vi "GameToIAState.vi"(8 "error in (no error)":errorcluster, 11 "Game in":refnum<class "Game.lvclass">) -> (0 "error out":errorcluster, 2 "IA State out":T1={"our_robots"=[], "enemy_robots"=[], "balls"=[], "geometry"={"line_width"=0, "field_length"=0, "field_width"=0, "boundary_width"=0, "referee_width"=0, "goal_width"=0, "goal_depth"=0, "goal_wall_width"=0, "center_circle_radius"=0, "defense_radius"=0, "defense_stretch"=0, "free_kick_from_defense_dist"=0, "penalty_spot_from_field_line_dist"=0, "penalty_line_from_spot_dist"=0}, "IA Judge"={"stage"="", "command"="", "our_goalie_id"=0.0, "enemy_goalie_id"=0.0, "command enum"=enum."Halt", "Time"=enum."Azul"}, "Received Timestamp"=timestamp(0 s since 1904-01-01), "Events"={"Touch"=FALSE, "Ball out"=FALSE, "id touch"=0.0, "Ball out of \nVision"=FALSE, "Ball inside \nGoalie area"=FALSE, "Robot not responding"=FALSE, "Robots responding status"=[1.0, 1.0, 1.0, 1.0, 1.0, 1.0], "Enemy Ball \nPossession"=FALSE, "Pass State"=FALSE, "id end of pass"=0.0, "Kick"=FALSE, "Id ini Possession"=0.0, "Ball Possesion"=FALSE, "Id Possesion"=0.0, "Direct Kick"=FALSE, "2nd Strk Ativo"=FALSE}}, 3 "Game out":refnum<class "Game.lvclass">)   [LabVIEW 2023, in "Game.lvclass"]
uses:
  Game.lvclass
  Vision_class/Old vision/SSL Detection Frame Simple Estimator Cameras VelCmd Folder/Core/AI Input.ctl
  Vision_class/Old vision/Controls/AI Robot.ctl
  Vision_class/Old vision/Controls/Functions Enum.ctl
  Vision_class/Old vision/Controls/AttackerStates.ctl
  Vision_class/Old vision/Controls/PathDests.ctl
  Vision_class/Old vision/Controls/PathDest.ctl
  Navigation/VSSNavigation/VSSAttackerStates.ctl
  Vision_class/Old vision/SSL Detection Frame Simple Estimator Cameras VelCmd Folder/Core/AI Ball.ctl
  Vision_class/Old vision/SSL Detection Frame Simple Estimator Cameras VelCmd Folder/Core/Field Size.ctl
  Vision_class/Old vision/SSL Detection Frame Simple Estimator Cameras VelCmd Folder/Core/AI Judge.ctl
  Communication_class/Paths/MessageAI_State Folder/Intel/Command Enum.ctl
  Vision_class/Old vision/SSL Detection Frame Simple Estimator Cameras VelCmd Folder/Util/Events/Events.ctl
  Game.lvclass/Game.ctl
  Team_class/Team.lvclass/Team.ctl
  Object_class/Object.lvclass/Object.ctl
  Ball_class/Ball.lvclass/Ball.ctl
  Events_class/Events.lvclass/Events.ctl
  Referee_class/Referee.lvclass/Referee.ctl
  Robot_class/Robot.lvclass/Robot.ctl
  Robot_class/Read id.vi
  Object_class/Read x.vi
  Object_class/Read y.vi
  Robot_class/Read orientation.vi
  Robot_class/Read dribble.vi
  Robot_class/Read est_v_tang.vi
  Robot_class/Read est_v_norm.vi
  Object_class/Read pos_est_x.vi
  Object_class/Read pos_est_y.vi
  Robot_class/Read path.vi
  Robot_class/Read path_smooth.vi
  Robot_class/Read dest_x.vi
  Robot_class/Read dest_y.vi
  Robot_class/Read dest_orientation.vi
  Robot_class/Read v_ang.vi
  Robot_class/Read v_norm.vi
  Robot_class/Read v_tang.vi
  Read DefensiveTeam.vi
  Read OffensiveTeam.vi
  Read KeeperTeam.vi
  Read EnemyRef.vi
  Read BallRef.vi
  Read EventsRef.vi
  Read FieldRef.vi
  Read Referee.vi
  Read TimeRef.vi
  Read NavigationTeam.vi
  Team_class/Read RobotRef.vi
  Referee_class/Read command_from_referee.vi
  Referee_class/Read command_interpreted.vi
  Events_class/Read ball_inside_enemy_goalie_area.vi
  Events_class/Read ball_inside_our_goalie_area.vi
  Events_class/Read ball_out.vi
  Events_class/Read ball_out_of_vision.vi
  Events_class/Read enemy_ball_possesion.vi
  Events_class/Read id_enemy_ball_possesion.vi
  Events_class/Read id_our_balll_possesion.vi
  Events_class/Read id_touch.vi
  Events_class/Read kick.vi
  Events_class/Read our_balll_possesion.vi
  Events_class/Read touch.vi
  Ball_class/Read v_x.vi
  Ball_class/Read v_y.vi
  Ally_class/Ally.lvclass
  C:/Users/roboi/Downloads/VSS_AI-Larc2023/Team_class/Team.lvclass
  Robot_class/Robot.lvclass
  C:/Users/roboi/Downloads/VSS_AI-Larc2023/Object_class/Object.lvclass
  Ball_class/Ball.lvclass
  Enemy_class/Enemy.lvclass
  Events_class/Events.lvclass
  Field_class/Field.lvclass
  Referee_class/Referee.lvclass
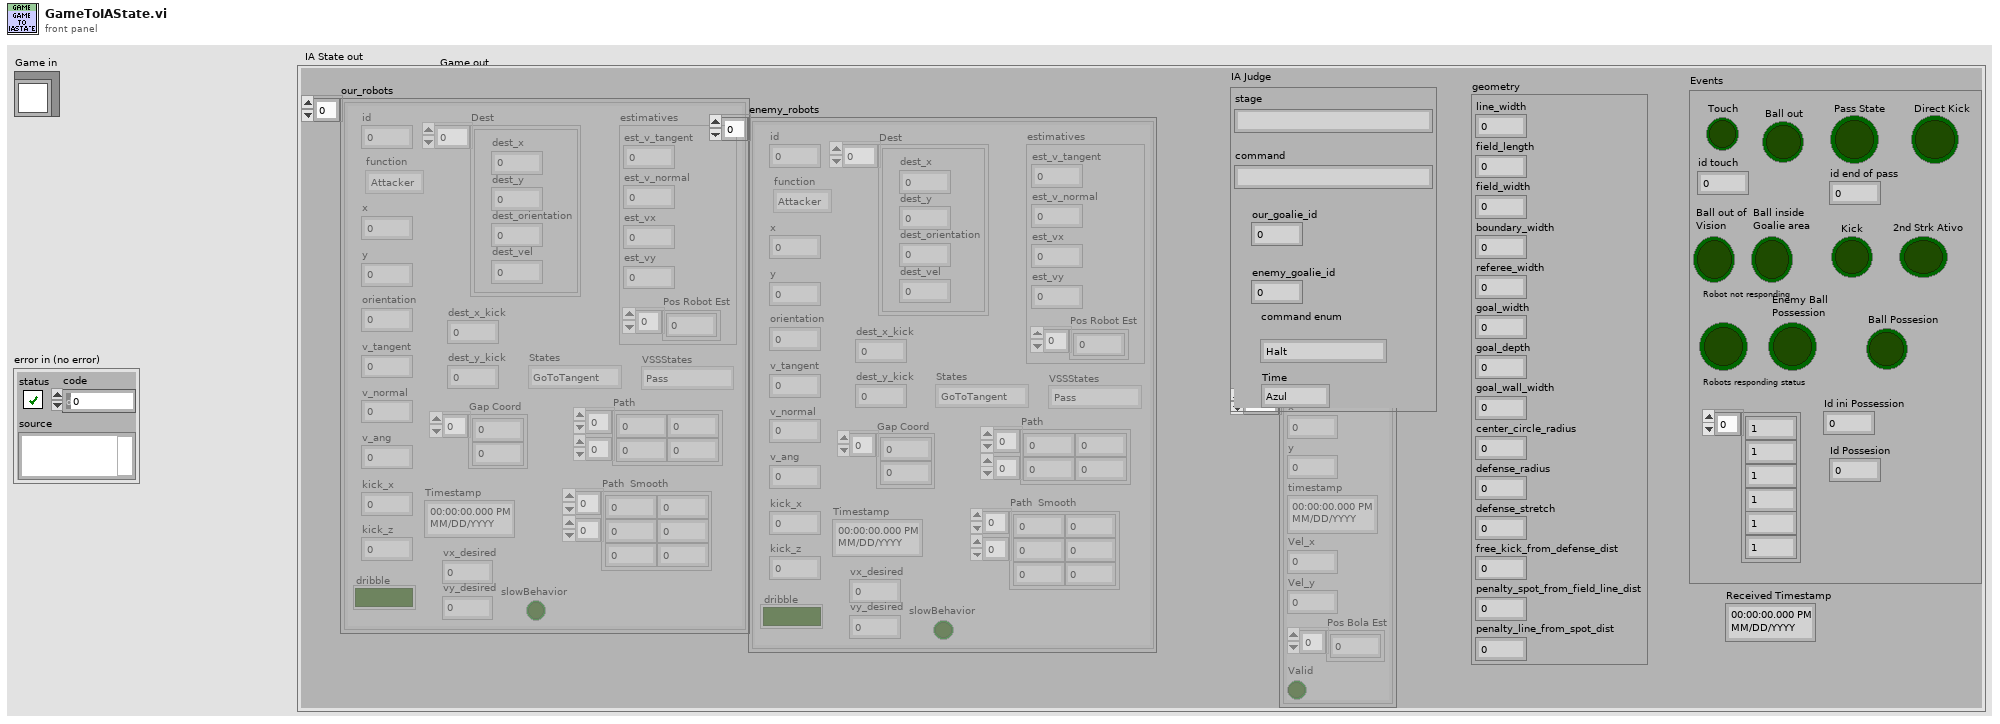
[diagram p1: front panel]
types:
  T1 = typedef "AI Input.ctl" = cluster{"our_robots":T2[], "enemy_robots":T2[], "balls":T8[], "geometry":T9, "IA Judge":T10, "Received Timestamp":timestamp, "Events":T12}
  T2 = typedef "AI Robot.ctl" = cluster{"id":u32, "function":T3, "x":dbl, "y":dbl, "orientation":dbl, "v_tangent":dbl, "v_normal":dbl, "v_ang":dbl, "kick_x":dbl, "kick_z":dbl, "dribble":bool, "Timestamp":timestamp, "estimatives":cluster{"est_v_tangent":dbl, "est_v_normal":dbl, "est_vx":dbl, "est_vy":dbl, "Pos Robot Est":dbl[]}, "dest_x_kick":dbl, "dest_y_kick":dbl, "Gap Coord":dbl[], "States":T4, "Path ":dbl[][], "Path  Smooth":dbl[][], "Dest":T5, "vx_desired":dbl, "vy_desired":dbl, "slowBehavior":bool, "VSSStates":T7}
  T3 = typedef "Functions Enum.ctl" = enum16{"2nd Striker", "Attacker", "Goalie", "Defender", "Striker", "Goto 0", "Dummy", "Kicker", "ZigZag 0", "ZigZag 1", "ZigZag 2", "ZigZag 3", "ZigZag 4", "ZigZag 5", "ZigZag 6", "ZigZag 7", "ZigZag 8", ""}
  T4 = typedef "AttackerStates.ctl" = enum16{"Pass", "GoToTangent", "BallGetting", "GoToKick", ""}
  T5 = typedef "PathDests.ctl" = T6[]
  T6 = typedef "PathDest.ctl" = cluster{"dest_x":dbl, "dest_y":dbl, "dest_orientation":dbl, "dest_vel":dbl}
  T7 = typedef "VSSAttackerStates.ctl" = enum16{"Pass", "GoToTangent", "BallGetting", "GoToKick", "Rotate anti-clockwise", "Rotate Clockwise", ""}
  T8 = typedef "AI Ball.ctl" = cluster{"x":dbl, "y":dbl, "timestamp":timestamp, "Vel_x":dbl, "Vel_y":dbl, "Pos Bola Est":dbl[], "Valid":bool}
  T9 = typedef "Field Size.ctl" = cluster{"line_width":u32, "field_length":u32, "field_width":u32, "boundary_width":u32, "referee_width":u32, "goal_width":u32, "goal_depth":u32, "goal_wall_width":u32, "center_circle_radius":u32, "defense_radius":u32, "defense_stretch":u32, "free_kick_from_defense_dist":u32, "penalty_spot_from_field_line_dist":u32, "penalty_line_from_spot_dist":u32}
  T10 = typedef "AI Judge.ctl" = cluster{"stage":string, "command":string, "our_goalie_id":dbl, "enemy_goalie_id":dbl, "command enum":T11, "Time":enum16{"Azul", "Amarelo"}}
  T11 = typedef "Command Enum.ctl" = enum16{"Halt", "Stop", "Force Start", "PKA Normal Start", "Prepare Kickoff Ally", "PKE Normal Start", "Prepare Kickoff Enemy", "Prepare Penalty Ally", "PPA Normal Start", "Prepare Penalty Enemy", "PPE Normal Start", "Direct Free Enemy", "Direct Free Ally", "Indirect Free Enemy", "Indirect Free Ally", "Timeout Enemy", "Timeout Ally", "Goal Enemy", "Goal Ally", "Ball Placement Enemy", "Ball Placement Ally", "Normal Half Time", "Extra Time Break", "Extra Half Time", "None", "Post Game"}
  T12 = typedef "Events.ctl" = cluster{"Touch":bool, "Ball out":bool, "id touch":dbl, "Ball out of \nVision":bool, "Ball inside \nGoalie area":bool, "Robot not responding":bool, "Robots responding status":dbl[], "Enemy Ball \nPossession":bool, "Pass State":bool, "id end of pass":dbl, "Kick":bool, "Id ini Possession":dbl, "Ball Possesion":bool, "Id Possesion":dbl, "Direct Kick":bool, "2nd Strk Ativo":bool}
  T13 = typedef "command_interpreted.ctl" = enum16{"Goal Ally", "Goal Enemy", "Ball Placement Enemy", "Ball Placement Ally", "Normal Half Time", "Extra Time  Break", "Extra Half Time", "None", "Post Game", "PKA Normal Start", "Prepare Kickoff Ally", "PKE Normal Start", "Prepare Kickoff Enemy", "Force Start", "Halt", "Timeout", "Prepare Penalty Ally", "Prepare Penalty Enemy", "PPA NormalStart", "PPE Normal Start", "Indirect Free Ally", "Direct Free Enemy", "Direct Free Ally", "Indirect Free Enemy", "Stop"}
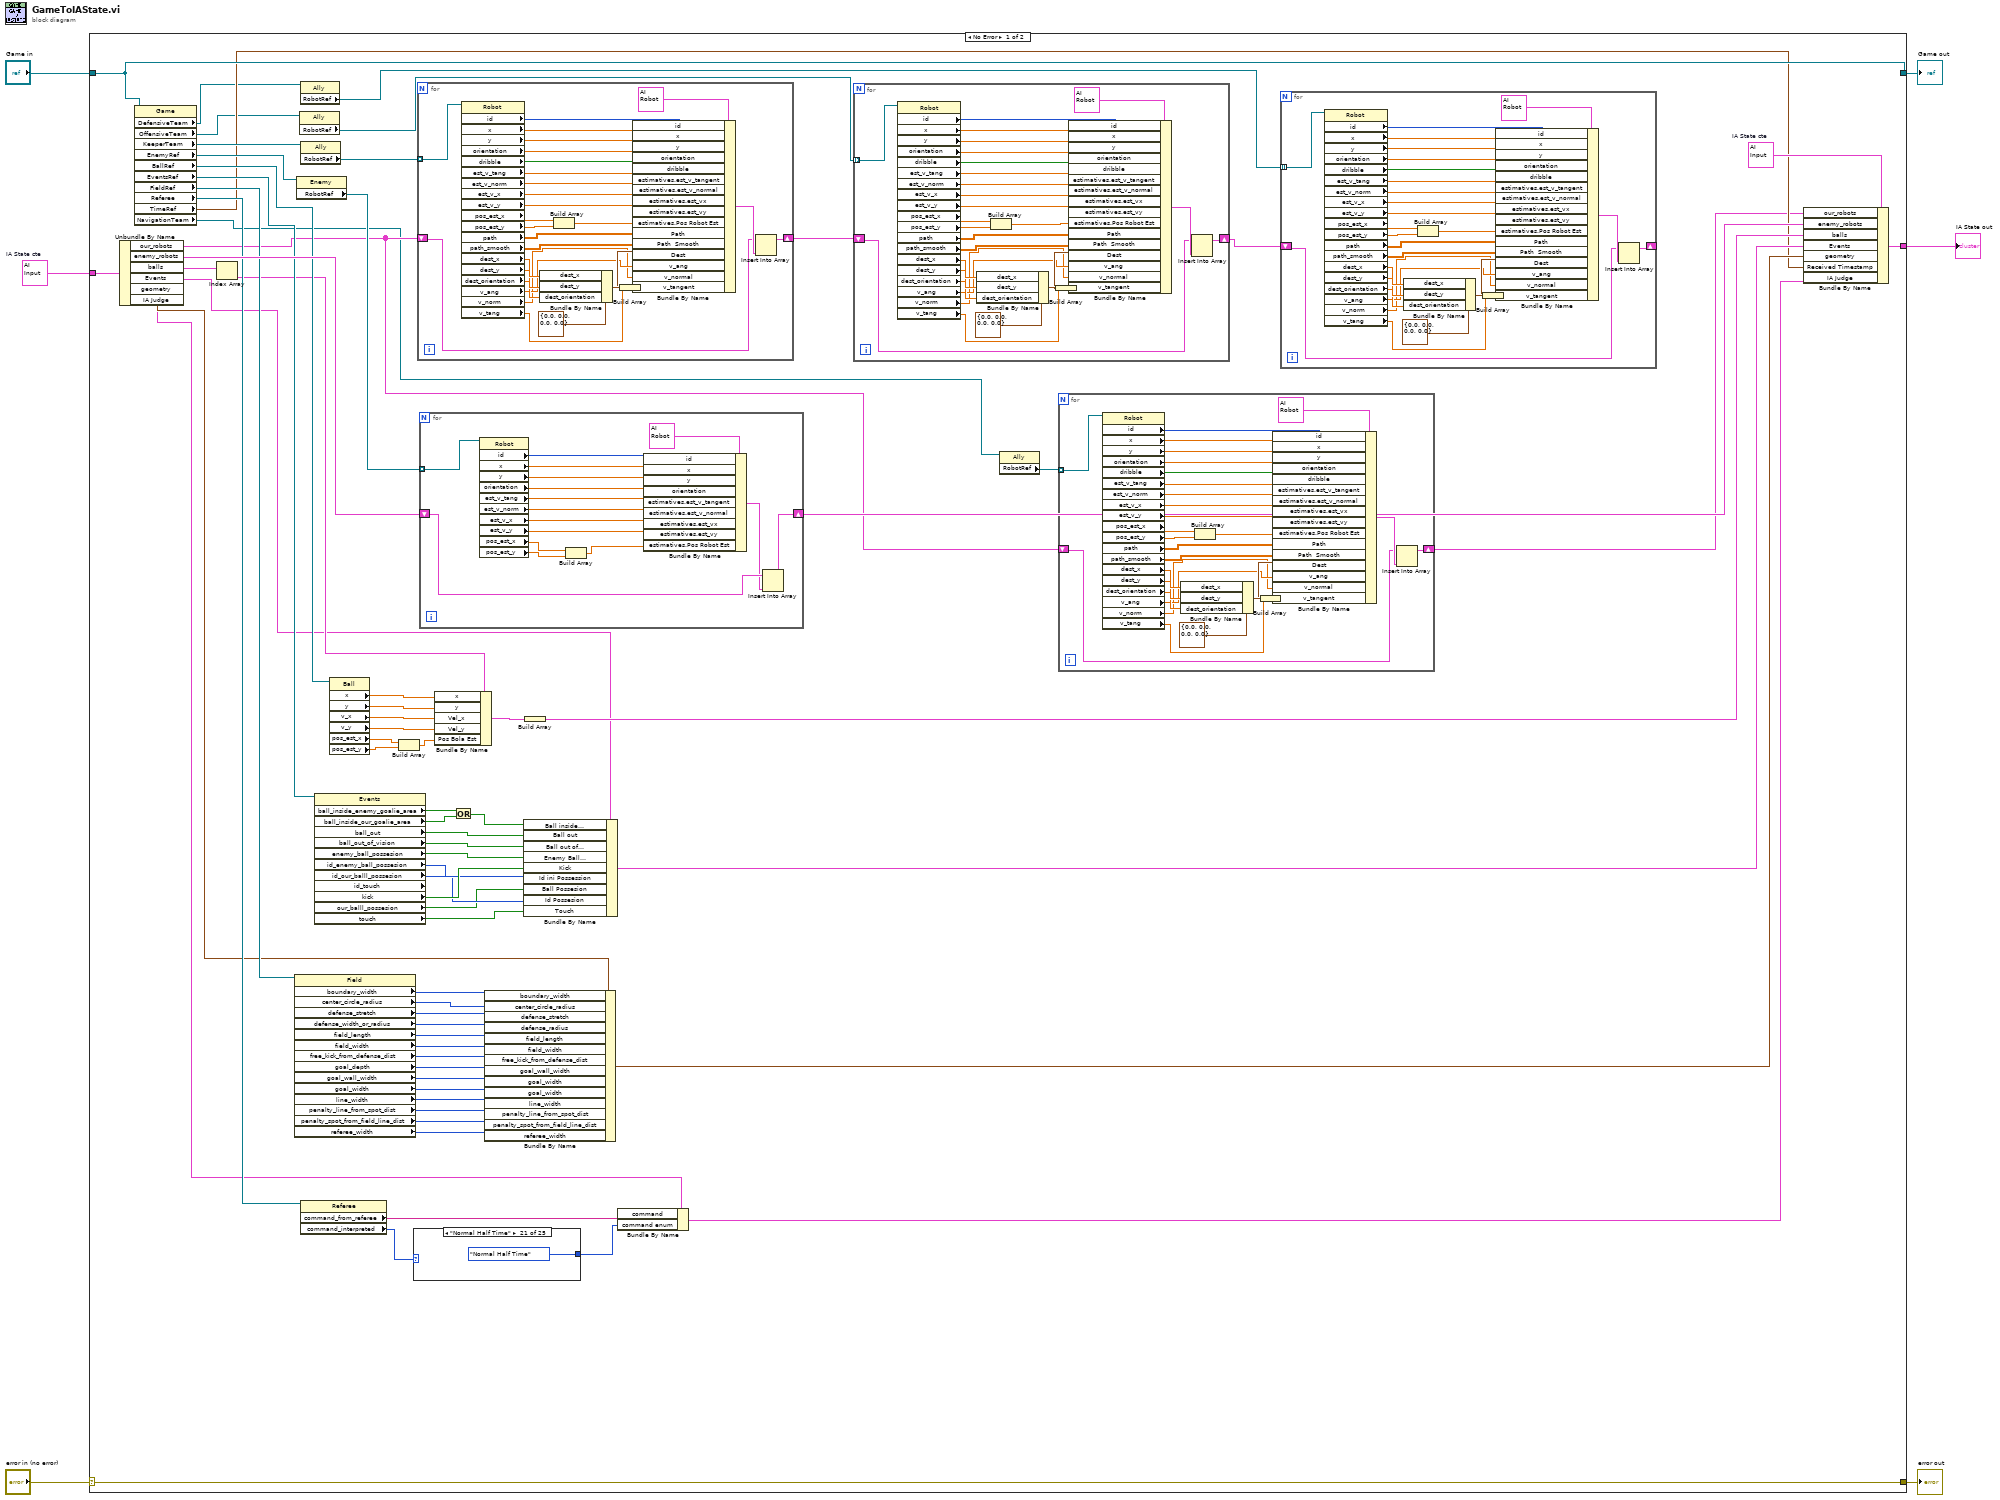
[diagram p0: block diagram]
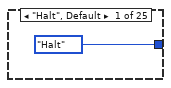
[diagram p2: hidden frame]
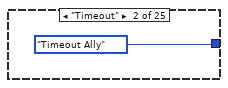
[diagram p3: hidden frame]
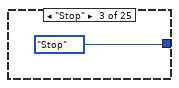
[diagram p4: hidden frame]
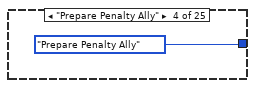
[diagram p5: hidden frame]
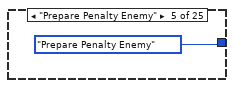
[diagram p6: hidden frame]
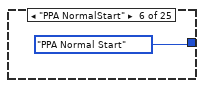
[diagram p7: hidden frame]
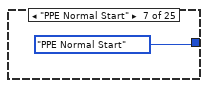
[diagram p8: hidden frame]
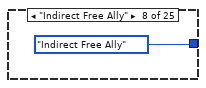
[diagram p9: hidden frame]
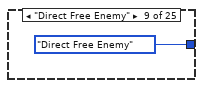
[diagram p10: hidden frame]
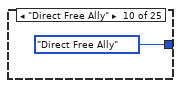
[diagram p11: hidden frame]
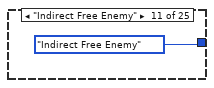
[diagram p12: hidden frame]
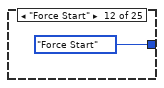
[diagram p13: hidden frame]
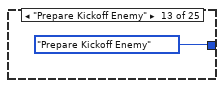
[diagram p14: hidden frame]
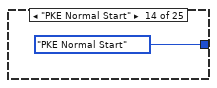
[diagram p15: hidden frame]
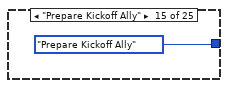
[diagram p16: hidden frame]
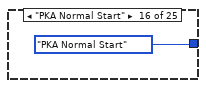
[diagram p17: hidden frame]
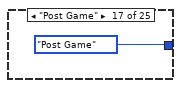
[diagram p18: hidden frame]
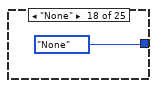
[diagram p19: hidden frame]
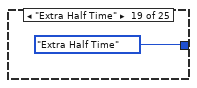
[diagram p20: hidden frame]
diagram:
  w2 = T1 {"our_robots"=[], "enemy_robots"=[], "balls"=[], "geometry"={"line_width"=0, "field_length"=0, "field_width"=0, "boundary_width"=0, "referee_width"=0, "goal_width"=0, "goal_depth"=0, "goal_wall_width"=0, "center_circle_radius"=0, "defense_radius"=0, "defense_stretch"=0, "free_kick_from_defense_dist"=0, "penalty_spot_from_field_line_dist"=0, "penalty_line_from_spot_dist"=0}, "IA Judge"={"stage"="", "command"="", "our_goalie_id"=0.0, "enemy_goalie_id"=0.0, "command enum"=enum."Halt", "Time"=enum."Azul"}, "Received Timestamp"=timestamp(0 s since 1904-01-01), "Events"={"Touch"=FALSE, "Ball out"=FALSE, "id touch"=0.0, "Ball out of \nVision"=FALSE, "Ball inside \nGoalie area"=FALSE, "Robot not responding"=FALSE, "Robots responding status"=[], "Enemy Ball \nPossession"=FALSE, "Pass State"=FALSE, "id end of pass"=0.0, "Kick"=FALSE, "Id ini Possession"=0.0, "Ball Possesion"=FALSE, "Id Possesion"=0.0, "Direct Kick"=FALSE, "2nd Strk Ativo"=FALSE}}  # IA State cte
  n1 = case shown="No Error" "error in (no error)" {
    selector: "error in (no error)" -> [w77 w233]
    tunnel: [w77 w233] -> w5
    tunnel: [w76 w232] -> w3
    tunnel: "Game in" -> [w76 w232]
    tunnel: w2 -> [w71 w231]
    tunnel: [w17 w231] -> w1
    frame No Error {
      w68 = T1 {"our_robots"=[], "enemy_robots"=[], "balls"=[], "geometry"={"line_width"=0, "field_length"=0, "field_width"=0, "boundary_width"=0, "referee_width"=0, "goal_width"=0, "goal_depth"=0, "goal_wall_width"=0, "center_circle_radius"=0, "defense_radius"=0, "defense_stretch"=0, "free_kick_from_defense_dist"=0, "penalty_spot_from_field_line_dist"=0, "penalty_line_from_spot_dist"=0}, "IA Judge"={"stage"="", "command"="", "our_goalie_id"=0.0, "enemy_goalie_id"=0.0, "command enum"=enum."Halt", "Time"=enum."Azul"}, "Received Timestamp"=timestamp(0 s since 1904-01-01), "Events"={"Touch"=FALSE, "Ball out"=FALSE, "id touch"=0.0, "Ball out of \nVision"=FALSE, "Ball inside \nGoalie area"=FALSE, "Robot not responding"=FALSE, "Robots responding status"=[], "Enemy Ball \nPossession"=FALSE, "Pass State"=FALSE, "id end of pass"=0.0, "Kick"=FALSE, "Id ini Possession"=0.0, "Ball Possesion"=FALSE, "Id Possesion"=0.0, "Direct Kick"=FALSE, "2nd Strk Ativo"=FALSE}}  # IA State cte
      n2 = Unbundle By Name(w71) -> ("our_robots"=w10:T2[], "enemy_robots"=w70:T2[], "balls"=w26:T8[], "Events"=w24:T12, "geometry"=w23:T9, "IA Judge"=w21:T10)
      n3 = property class="Game"(reference=w76) -> ("DefensiveTeam"=w15:refnum<class "Ally.lvclass">, "OffensiveTeam"=w16:refnum<class "Ally.lvclass">, "KeeperTeam"=w75:refnum<class "Ally.lvclass">, "EnemyRef"=w73:refnum<class "Enemy.lvclass">, "BallRef"=w69:refnum<class "Ball.lvclass">, "EventsRef"=w57:refnum<class "Events.lvclass">, "FieldRef"=w44:refnum<class "Field.lvclass">, "Referee"=w28:refnum<class "Referee.lvclass">, "TimeRef"=w22:timestamp, "NavigationTeam"=w8:refnum<class "Ally.lvclass">)  [unwired: 1 in, 2 out]
      n4 = Index Array(array=w26) -> (element=w25:T8)  [unwired: 1 in]
      n5 = property class="Field"(reference=w44) -> ("boundary_width"=w43:i32, "center_circle_radius"=w42:i32, "defense_stretch"=w41:i32, "defense_width_or_radius"=w40:i32, "field_length"=w39:i32, "field_width"=w38:i32, "free_kick_from_defense_dist"=w37:i32, "goal_depth"=w36:i32, "goal_wall_width"=w35:i32, "goal_width"=w34:i32, "line_width"=w33:i32, "penalty_line_from_spot_dist"=w32:i32, "penalty_spot_from_field_line_dist"=w31:i32, "referee_width"=w30:i32)  [unwired: 1 in, 2 out]
      n6 = property class="Enemy"(reference=w73) -> ("RobotRef"=w72:refnum<class "Robot.lvclass">[])  [unwired: 1 in, 2 out]
      n7 = property class="Ally"(reference=w16) -> ("RobotRef"=w13:refnum<class "Robot.lvclass">[])  [unwired: 1 in, 2 out]
      n8 = property class="Ally"(reference=w15) -> ("RobotRef"=w14:refnum<class "Robot.lvclass">[])  [unwired: 1 in, 2 out]
      n9 = property class="Ally"(reference=w75) -> ("RobotRef"=w74:refnum<class "Robot.lvclass">[])  [unwired: 1 in, 2 out]
      n10 = property class="Referee"(reference=w28) -> ("command_from_referee"=w27:string, "command_interpreted"=w20:T13)  [unwired: 1 in, 2 out]
      n11 = property class="Events" props=["ball_inside_enemy_goalie_area", "ball_inside_our_goalie_area", "ball_out", "ball_out_of_vision", "enemy_ball_possesion", "id_enemy_ball_possesion", "id_our_balll_possesion", "id_touch", "kick", "our_balll_possesion", "touch"](reference=w57) -> ("ball_inside_enemy_goalie_area"=w55:bool, "ball_inside_our_goalie_area"=w56:bool, "ball_out"=w53:bool, "ball_out_of_vision"=w52:bool, "enemy_ball_possesion"=w51:bool, "id_enemy_ball_possesion"=w49:i32, "id_our_balll_possesion"=w48:i32, "kick"=w50:bool, "our_balll_possesion"=w47:bool, "touch"=w46:bool)  [unwired: 1 in, 3 out]
      n12 = property class="Ball"(reference=w69) -> ("x"=w66:dbl, "y"=w65:dbl, "v_x"=w64:dbl, "v_y"=w63:dbl, "pos_est_x"=w62:dbl, "pos_est_y"=w61:dbl)  [unwired: 1 in, 2 out]
      n13 = Build Array(w62, w61) -> (w60:dbl[])
      n14 = case shown="\"Normal Half Time\"" w20 {
        tunnel: [Command_Enum."Halt" ("command enum") Command_Enum."Timeout Ally" ("command enum") Command_Enum."Stop" ("command enum") Command_Enum."Prepare Penalty Ally" ("command enum") Command_Enum."Prepare Penalty Enemy" ("command enum") Command_Enum."PPA Normal Start" ("command enum") Command_Enum."PPE Normal Start" ("command enum") Command_Enum."Indirect Free Ally" ("command enum") Command_Enum."Direct Free Enemy" ("command enum") Command_Enum."Direct Free Ally" ("command enum") Command_Enum."Indirect Free Enemy" ("command enum") Command_Enum."Force Start" ("command enum") Command_Enum."Prepare Kickoff Enemy" ("command enum") Command_Enum."PKE Normal Start" ("command enum") Command_Enum."Prepare Kickoff Ally" ("command enum") Command_Enum."PKA Normal Start" ("command enum") Command_Enum."Post Game" ("command enum") Command_Enum."None" ("command enum") Command_Enum."Extra Half Time" ("command enum") Command_Enum."Extra Time Break" ("command enum") Command_Enum."Normal Half Time" ("command enum") Command_Enum."Ball Placement Ally" ("command enum") Command_Enum."Ball Placement Enemy" ("command enum") Command_Enum."Goal Enemy" ("command enum") Command_Enum."Goal Ally" ("command enum")] -> w19
        frame "Halt", Default {
        }
        frame "Timeout" {
        }
        frame "Stop" {
        }
        frame "Prepare Penalty Ally" {
        }
        frame "Prepare Penalty Enemy" {
        }
        frame "PPA NormalStart" {
        }
        frame "PPE Normal Start" {
        }
        frame "Indirect Free Ally" {
        }
        frame "Direct Free Enemy" {
        }
        frame "Direct Free Ally" {
        }
        frame "Indirect Free Enemy" {
        }
        frame "Force Start" {
        }
        frame "Prepare Kickoff Enemy" {
        }
        frame "PKE Normal Start" {
        }
        frame "Prepare Kickoff Ally" {
        }
        frame "PKA Normal Start" {
        }
        frame "Post Game" {
        }
        frame "None" {
        }
        frame "Extra Half Time" {
        }
        frame "Extra Time  Break" {
        }
        frame "Normal Half Time" {
        }
        frame "Ball Placement Ally" {
        }
        frame "Ball Placement Enemy" {
        }
        frame "Goal Enemy" {
        }
        frame "Goal Ally" {
        }
      }
      n15 = for {
        tunnel: w74 -> [w210] mode=indexing
        shift-right: [w211] -> w12
        shift-left: w10 -> [w212]
        n16 = property class="Robot"(reference=w210) -> ("id"=w209:i32, "x"=w208:dbl, "y"=w207:dbl, "orientation"=w206:dbl, "dribble"=w205:bool, "est_v_tang"=w204:dbl, "est_v_norm"=w203:dbl, "est_v_x"=w202:dbl, "est_v_y"=w201:dbl, "pos_est_x"=w200:dbl, "pos_est_y"=w199:dbl, "path"=w197:dbl[][], "path_smooth"=w196:dbl[][], "dest_x"=w195:dbl, "dest_y"=w194:dbl, "dest_orientation"=w193:dbl, "v_ang"=w189:dbl, "v_norm"=w188:dbl, "v_tang"=w187:dbl)  [unwired: 1 in, 2 out]
        n17 = Bundle By Name(cluster=T6 {"dest_x"=0.0, "dest_y"=0.0, "dest_orientation"=0.0, "dest_vel"=0.0} ("element"), "dest_x"=w195, "dest_y"=w194, "dest_orientation"=w193) -> (w191:T6)
        n18 = Build Array(w200, w199) -> (w198:dbl[])
        n19 = Build Array(w191) -> (w190:T6[])
        n20 = Bundle By Name(cluster=T2 {"id"=0, "function"=enum."Attacker", "x"=0.0, "y"=0.0, "orientation"=0.0, "v_tangent"=0.0, "v_normal"=0.0, "v_ang"=0.0, "kick_x"=0.0, "kick_z"=0.0, "dribble"=FALSE, "Timestamp"=timestamp(0 s since 1904-01-01), "estimatives"={"est_v_tangent"=0.0, "est_v_normal"=0.0, "est_vx"=0.0, "est_vy"=0.0, "Pos Robot Est"=[]}, "dest_x_kick"=0.0, "dest_y_kick"=0.0, "Gap Coord"=[], "States"=enum."GoToTangent", "Path "=[], "Path  Smooth"=[], "Dest"=[], "vx_desired"=0.0, "vy_desired"=0.0, "slowBehavior"=FALSE, "VSSStates"=enum."Pass"} ("Robot"), "id"=w209, "x"=w208, "y"=w207, "orientation"=w206, "dribble"=w205, "estimatives.est_v_tangent"=w204, "estimatives.est_v_normal"=w203, "estimatives.est_vx"=w202, "estimatives.est_vy"=w201, "estimatives.Pos Robot Est"=w198, "Path"=w197, "Path  Smooth"=w196, "Dest"=w190, "v_ang"=w189, "v_normal"=w188, "v_tangent"=w187) -> (w213:T2)
        n21 = Insert Into Array(array=w212, new element=w213) -> (w211:T2[])  [unwired: 1 in]
      }
      n22 = for {
        tunnel: w72 -> [w225] mode=indexing
        shift-right: [w215] -> w67
        shift-left: w70 -> [w224]
        n23 = property class="Robot"(reference=w225) -> ("id"=w227:i32, "x"=w228:dbl, "y"=w229:dbl, "orientation"=w230:dbl, "est_v_tang"=w223:dbl, "est_v_norm"=w222:dbl, "est_v_x"=w221:dbl, "est_v_y"=w220:dbl, "pos_est_x"=w219:dbl, "pos_est_y"=w218:dbl)  [unwired: 1 in, 2 out]
        n24 = Build Array(w219, w218) -> (w217:dbl[])
        n25 = Bundle By Name(cluster=T2 {"id"=0, "function"=enum."Attacker", "x"=0.0, "y"=0.0, "orientation"=0.0, "v_tangent"=0.0, "v_normal"=0.0, "v_ang"=0.0, "kick_x"=0.0, "kick_z"=0.0, "dribble"=FALSE, "Timestamp"=timestamp(0 s since 1904-01-01), "estimatives"={"est_v_tangent"=0.0, "est_v_normal"=0.0, "est_vx"=0.0, "est_vy"=0.0, "Pos Robot Est"=[]}, "dest_x_kick"=0.0, "dest_y_kick"=0.0, "Gap Coord"=[], "States"=enum."GoToTangent", "Path "=[], "Path  Smooth"=[], "Dest"=[], "vx_desired"=0.0, "vy_desired"=0.0, "slowBehavior"=FALSE, "VSSStates"=enum."Pass"} ("Robot"), "id"=w227, "x"=w228, "y"=w229, "orientation"=w230, "estimatives.est_v_tangent"=w223, "estimatives.est_v_normal"=w222, "estimatives.est_vx"=w221, "estimatives.est_vy"=w220, "estimatives.Pos Robot Est"=w217) -> (w216:T2)
        n26 = Insert Into Array(array=w224, new element=w216) -> (w215:T2[])  [unwired: 1 in]
      }
      n27 = Bundle By Name(cluster=w25, "x"=w66, "y"=w65, "Vel_x"=w64, "Vel_y"=w63, "Pos Bola Est"=w60) -> (w59:T8)
      n28 = Or(x=w55, y=w56) -> (x .or. y?=w54:bool)
      n29 = Bundle By Name(cluster=w23, "boundary_width"=w43, "center_circle_radius"=w42, "defense_stretch"=w41, "defense_radius"=w40, "field_length"=w39, "field_width"=w38, "free_kick_from_defense_dist"=w37, "goal_wall_width"=w36, "goal_width"=w35, "goal_width"=w34, "line_width"=w33, "penalty_line_from_spot_dist"=w32, "penalty_spot_from_field_line_dist"=w31, "referee_width"=w30) -> (w29:T9)
      n30 = Bundle By Name(cluster=w24, "Ball inside \nGoalie area"=w54, "Ball out"=w53, "Ball out of \nVision"=w52, "Enemy Ball \nPossession"=w51, "Kick"=w50, "Id ini Possession"=w49, "Ball Possesion"=w47, "Id Possesion"=w48, "Touch"=w46) -> (w45:T12)
      n31 = Build Array(w59) -> (w58:T8[])
      n32 = Bundle By Name(cluster=w21, "command"=w27, "command enum"=w19) -> (w18:T10)
      n33 = for {
        tunnel: w13 -> [w157] mode=indexing
        shift-right: [w158] -> w11
        shift-left: w12 -> [w159]
        n34 = property class="Robot"(reference=w157) -> ("id"=w156:i32, "x"=w155:dbl, "y"=w154:dbl, "orientation"=w153:dbl, "dribble"=w152:bool, "est_v_tang"=w151:dbl, "est_v_norm"=w150:dbl, "est_v_x"=w149:dbl, "est_v_y"=w148:dbl, "pos_est_x"=w147:dbl, "pos_est_y"=w146:dbl, "path"=w144:dbl[][], "path_smooth"=w143:dbl[][], "dest_x"=w142:dbl, "dest_y"=w141:dbl, "dest_orientation"=w140:dbl, "v_ang"=w136:dbl, "v_norm"=w135:dbl, "v_tang"=w134:dbl)  [unwired: 1 in, 2 out]
        n35 = Bundle By Name(cluster=T6 {"dest_x"=0.0, "dest_y"=0.0, "dest_orientation"=0.0, "dest_vel"=0.0} ("element"), "dest_x"=w142, "dest_y"=w141, "dest_orientation"=w140) -> (w138:T6)
        n36 = Build Array(w147, w146) -> (w145:dbl[])
        n37 = Build Array(w138) -> (w137:T6[])
        n38 = Bundle By Name(cluster=T2 {"id"=0, "function"=enum."Attacker", "x"=0.0, "y"=0.0, "orientation"=0.0, "v_tangent"=0.0, "v_normal"=0.0, "v_ang"=0.0, "kick_x"=0.0, "kick_z"=0.0, "dribble"=FALSE, "Timestamp"=timestamp(0 s since 1904-01-01), "estimatives"={"est_v_tangent"=0.0, "est_v_normal"=0.0, "est_vx"=0.0, "est_vy"=0.0, "Pos Robot Est"=[]}, "dest_x_kick"=0.0, "dest_y_kick"=0.0, "Gap Coord"=[], "States"=enum."GoToTangent", "Path "=[], "Path  Smooth"=[], "Dest"=[], "vx_desired"=0.0, "vy_desired"=0.0, "slowBehavior"=FALSE, "VSSStates"=enum."Pass"} ("Robot"), "id"=w156, "x"=w155, "y"=w154, "orientation"=w153, "dribble"=w152, "estimatives.est_v_tangent"=w151, "estimatives.est_v_normal"=w150, "estimatives.est_vx"=w149, "estimatives.est_vy"=w148, "estimatives.Pos Robot Est"=w145, "Path"=w144, "Path  Smooth"=w143, "Dest"=w137, "v_ang"=w136, "v_normal"=w135, "v_tangent"=w134) -> (w160:T2)
        n39 = Insert Into Array(array=w159, new element=w160) -> (w158:T2[])  [unwired: 1 in]
      }
      n40 = property class="Ally"(reference=w8) -> ("RobotRef"=w9:refnum<class "Robot.lvclass">[])  [unwired: 1 in, 2 out]
      n41 = for {
        tunnel: w9 -> [w101] mode=indexing
        shift-right: [w102] -> w7
        shift-left: w10 -> [w103]
        n42 = property class="Robot"(reference=w101) -> ("id"=w100:i32, "x"=w99:dbl, "y"=w98:dbl, "orientation"=w97:dbl, "dribble"=w96:bool, "est_v_tang"=w95:dbl, "est_v_norm"=w94:dbl, "est_v_x"=w93:dbl, "est_v_y"=w92:dbl, "pos_est_x"=w91:dbl, "pos_est_y"=w90:dbl, "path"=w88:dbl[][], "path_smooth"=w87:dbl[][], "dest_x"=w86:dbl, "dest_y"=w85:dbl, "dest_orientation"=w84:dbl, "v_ang"=w80:dbl, "v_norm"=w79:dbl, "v_tang"=w78:dbl)  [unwired: 1 in, 2 out]
        n43 = Bundle By Name(cluster=T6 {"dest_x"=0.0, "dest_y"=0.0, "dest_orientation"=0.0, "dest_vel"=0.0} ("element"), "dest_x"=w86, "dest_y"=w85, "dest_orientation"=w84) -> (w82:T6)
        n44 = Build Array(w91, w90) -> (w89:dbl[])
        n45 = Build Array(w82) -> (w81:T6[])
        n46 = Bundle By Name(cluster=T2 {"id"=0, "function"=enum."Attacker", "x"=0.0, "y"=0.0, "orientation"=0.0, "v_tangent"=0.0, "v_normal"=0.0, "v_ang"=0.0, "kick_x"=0.0, "kick_z"=0.0, "dribble"=FALSE, "Timestamp"=timestamp(0 s since 1904-01-01), "estimatives"={"est_v_tangent"=0.0, "est_v_normal"=0.0, "est_vx"=0.0, "est_vy"=0.0, "Pos Robot Est"=[]}, "dest_x_kick"=0.0, "dest_y_kick"=0.0, "Gap Coord"=[], "States"=enum."GoToTangent", "Path "=[], "Path  Smooth"=[], "Dest"=[], "vx_desired"=0.0, "vy_desired"=0.0, "slowBehavior"=FALSE, "VSSStates"=enum."Pass"} ("Robot"), "id"=w100, "x"=w99, "y"=w98, "orientation"=w97, "dribble"=w96, "estimatives.est_v_tangent"=w95, "estimatives.est_v_normal"=w94, "estimatives.est_vx"=w93, "estimatives.est_vy"=w92, "estimatives.Pos Robot Est"=w89, "Path"=w88, "Path  Smooth"=w87, "Dest"=w81, "v_ang"=w80, "v_normal"=w79, "v_tangent"=w78) -> (w104:T2)
        n47 = Insert Into Array(array=w103, new element=w104) -> (w102:T2[])  [unwired: 1 in]
      }
      n48 = for {
        tunnel: w14 -> [w129] mode=indexing
        shift-right: [w130] -> _
        shift-left: w11 -> [w131]
        n49 = property class="Robot"(reference=w129) -> ("id"=w128:i32, "x"=w127:dbl, "y"=w126:dbl, "orientation"=w125:dbl, "dribble"=w124:bool, "est_v_tang"=w123:dbl, "est_v_norm"=w122:dbl, "est_v_x"=w121:dbl, "est_v_y"=w120:dbl, "pos_est_x"=w119:dbl, "pos_est_y"=w118:dbl, "path"=w116:dbl[][], "path_smooth"=w115:dbl[][], "dest_x"=w114:dbl, "dest_y"=w113:dbl, "dest_orientation"=w112:dbl, "v_ang"=w108:dbl, "v_norm"=w107:dbl, "v_tang"=w106:dbl)  [unwired: 1 in, 2 out]
        n50 = Bundle By Name(cluster=T6 {"dest_x"=0.0, "dest_y"=0.0, "dest_orientation"=0.0, "dest_vel"=0.0} ("element"), "dest_x"=w114, "dest_y"=w113, "dest_orientation"=w112) -> (w110:T6)
        n51 = Build Array(w119, w118) -> (w117:dbl[])
        n52 = Build Array(w110) -> (w109:T6[])
        n53 = Bundle By Name(cluster=T2 {"id"=0, "function"=enum."Attacker", "x"=0.0, "y"=0.0, "orientation"=0.0, "v_tangent"=0.0, "v_normal"=0.0, "v_ang"=0.0, "kick_x"=0.0, "kick_z"=0.0, "dribble"=FALSE, "Timestamp"=timestamp(0 s since 1904-01-01), "estimatives"={"est_v_tangent"=0.0, "est_v_normal"=0.0, "est_vx"=0.0, "est_vy"=0.0, "Pos Robot Est"=[]}, "dest_x_kick"=0.0, "dest_y_kick"=0.0, "Gap Coord"=[], "States"=enum."GoToTangent", "Path "=[], "Path  Smooth"=[], "Dest"=[], "vx_desired"=0.0, "vy_desired"=0.0, "slowBehavior"=FALSE, "VSSStates"=enum."Pass"} ("Robot"), "id"=w128, "x"=w127, "y"=w126, "orientation"=w125, "dribble"=w124, "estimatives.est_v_tangent"=w123, "estimatives.est_v_normal"=w122, "estimatives.est_vx"=w121, "estimatives.est_vy"=w120, "estimatives.Pos Robot Est"=w117, "Path"=w116, "Path  Smooth"=w115, "Dest"=w109, "v_ang"=w108, "v_normal"=w107, "v_tangent"=w106) -> (w132:T2)
        n54 = Insert Into Array(array=w131, new element=w132) -> (w130:T2[])  [unwired: 1 in]
      }
      n55 = Bundle By Name(cluster=w68, "our_robots"=w7, "enemy_robots"=w67, "balls"=w58, "Events"=w45, "geometry"=w29, "Received Timestamp"=w22, "IA Judge"=w18) -> (w17:T1)
    }
    frame Error {
    }
  }
  "error out" <- w5
  "Game out" <- w3
  "IA State out" <- w1
